vi "util_file_write.vi"(8 "error in (no error)":errorcluster, 10 "string":string, 11 "config_path":path) -> (0 "error out":errorcluster)   [LabVIEW 2015, in "lv-build.lvlib"]
doc: "This VI will replace the contents of a file with the provided string. It will attempt to create or replace the file with the default permissions (read/write)."
uses:
  lv-build.lvlib
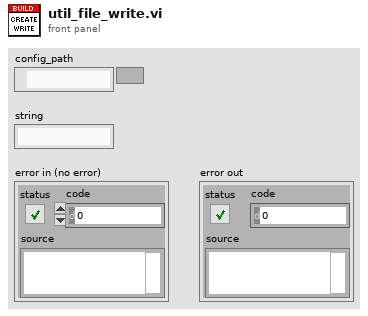
[diagram p1: front panel]
types:
  T1 = enum16{"open", "replace", "create", "open or create", "replace or create", "replace or create with confirmation"}
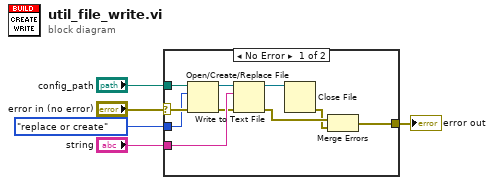
[diagram p0: block diagram]
diagram:
  n1 = case shown="No Error" "error in (no error)" {
    selector: "error in (no error)" -> [w8 w16]
    tunnel: [w15 w16] -> w5
    tunnel: "string" -> [w12 _]
    tunnel: "config_path" -> [w10 _]
    tunnel: T1."replace or create" ("operation (0:open)") -> [w6 _]
    frame No Error {
      n2 = Open/Create/Replace File(file path (use dialog)=w10, error in=w8, operation (0:open)=w6) -> (refnum out=w9:refnum<file>, error out=w7:errorcluster)  [unwired: 3 in, 1 out]
      n3 = Write to Text File(file (use dialog)=w9, text=w12, error in=w7) -> (refnum out=w13:refnum<file>, error out=w14:errorcluster)  [unwired: 1 in, 1 out]
      n4 = Close File(refnum=w13) -> (error out=w11:errorcluster)  [unwired: 1 in, 1 out]
      n5 = Merge Errors(w14, w11) -> (w15:errorcluster)
    }
    frame Error {
    }
  }
  "error out" <- w5
